vi "Add Element.vi"(8 "error in (no error)":errorcluster caption="错误输入（无错误）", 10 "迭代器.lvlib:雇员.lvclass":refnum<class "雇员.lvclass">, 11 "具体聚集 输入":refnum<class "具体聚集.lvclass"> caption="DNL_LabVIEW Object in") -> (0 "error out":errorcluster caption="错误输出", 3 "具体聚集 输出":refnum<class "具体聚集.lvclass"> caption="DNL_LabVIEW Object out")   [LabVIEW 2011, in "迭代器.lvlib" / "具体聚集.lvclass"]
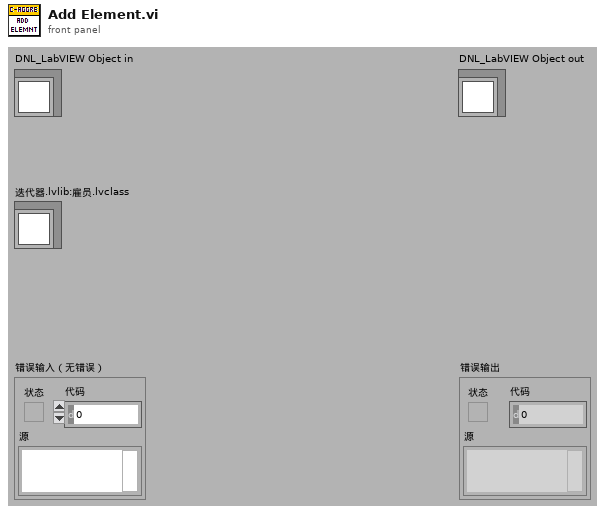
[diagram p1: front panel]
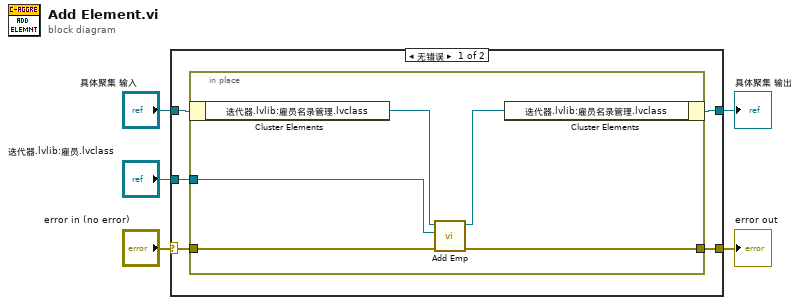
[diagram p0: block diagram]
diagram:
  n1 = case shown="无错误" "error in (no error)" {
    selector: "error in (no error)" -> [w9 w17]
    tunnel: [w6 w17] -> w4
    tunnel: "具体聚集 输入" -> [w8 w16]
    tunnel: "迭代器.lvlib:雇员.lvclass" -> [w10 _]
    tunnel: [w7 w16] -> w1
    frame No Error {
      n2 = in-place {
        in-place-border: w10 -> [w11]
        in-place-border: w9 -> [w13]
        in-place-border: [w12] -> w6
        n3 = in-place-cluster #1(w8) -> ("迭代器.lvlib:雇员名录管理.lvclass"=w15:refnum<class "雇员名录管理.lvclass">)
        n4 = call "Add Emp.vi"("error in (no error)"=w13, "迭代器.lvlib:雇员.lvclass"=w11, "雇员名录管理 输入"=w15) -> ("error out"=w12:errorcluster, "雇员名录管理 输出"=w14:refnum<class "雇员名录管理.lvclass">)  [unwired: 7 in]
        n5 = in-place-cluster #1("迭代器.lvlib:雇员名录管理.lvclass"=w14) -> (w7:refnum<class "具体聚集.lvclass">)
      }
    }
    frame Error {
    }
  }
  "error out" <- w4
  "具体聚集 输出" <- w1
